vi "Pre Enqueue Action.vi"(8 "error in (no error)":errorcluster, 10 "Message Array in":refnum<class "Message.lvclass">[](array[class]), 11 "Msg in":refnum<class "Cycle Msg.lvclass">) -> (0 "error out":errorcluster, 2 "Message Array out":refnum<class "Message.lvclass">[](array[class]))   [LabVIEW 2020, in "Sequencer.lvlib" / "Cycle Msg.lvclass"]
doc: "Action performed on the message array prior to the enqueue on the Sequencer Core.\n\nThis implementation re-enqueues the Cycle Msg at the end of the message array creating never ending execution cycle. An external interrupt is required to end the cycling."
uses:
  Cycle Msg.lvclass
  PPL/HDH.Actor Framework.Core.Actor.lvlibp/1abvi3w/vi.lib/ActorFramework/Message/Message.lvclass
  C:/Current projects/WS/PPL/HDH.Actor Framework.Core.Actor.lvlibp/1abvi3w/vi.lib/ActorFramework/Message/Message.lvclass
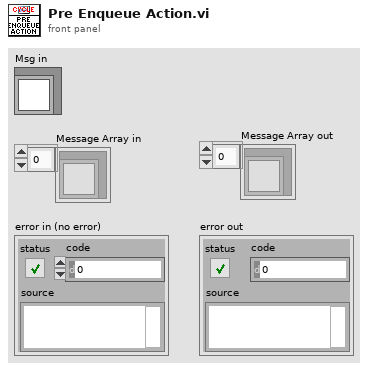
[diagram p1: front panel]
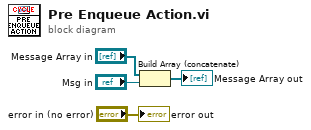
[diagram p0: block diagram]
diagram:
  n1 = Build Array (concatenate)("Message Array in", "Msg in") -> (→"Message Array out":refnum<class "Message.lvclass">[])
  "error out" <- "error in (no error)"
